vi "纳清pH电极校准.vi"() -> ()   [LabVIEW 2016, in "斯坦道多参数.lvlib"]
uses:
  <vilib>/Utility/miscctls.llb/LVPointTypeDef.ctl
  <vilib>/Analysis/NI_AALBase.lvlib
panel:
  out "滤波设定":sgl
  out "第二点信号值":dbl
  out "第一点信号值":dbl
  out "报警信息":string
  out "通讯状态":string
  out "第二点校准值":dbl
  out "第一点校准值":dbl
  in  "校准停止":bool
  in  "校准启动":bool
  in  "校准模式":u16(ring) items=["两点校准", "单点校准"]
  out "最小值":sgl format="%#.2f"
  out "最大值":sgl format="%#.2f"
  out "波形图表":dbl(graph) caption="历史曲线"
  out "mean":dbl caption="均值" format="%#.2f"
  out "standard deviation":dbl caption="标准差" format="%#.2f"
  out "变异系数":dbl format="%#.6f"
  out "测量值":sgl format="%#.2f"
  out "提示":string
  out "标液2":sgl
  out "标液1":sgl
  out "原始光强数值":sgl caption="信号值" format="%#.6f"
  out "温度":dbl format="%#.2f"
  # "pH电极设定"
  # "℃"
  # "mV"
  # "请选择校准模式:"
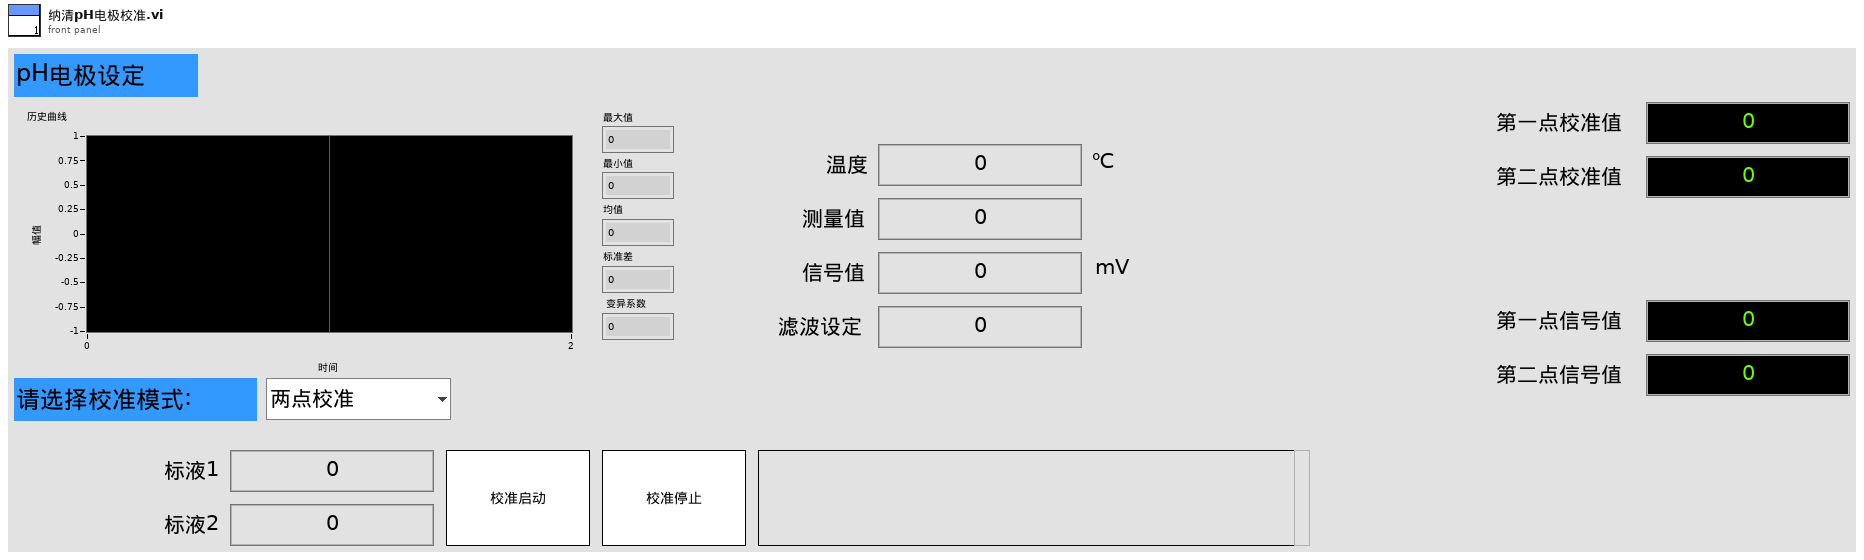
[diagram p1: front panel]
types:
  T1 = enum16{"pH", "DO", "Cond", "Turb", "ORP", "叶绿素a", "藻密度"}
  T2 = typedef "LVPointTypeDef.ctl" = cluster{"Horizontal":i16, "Vertical":i16}
  T3 = cluster{"报警码":u16, "pH数值":sgl, "0X0003_NC":sgl, "温度数据":sgl, "pH原始信号 mv":sgl, "0X0009_NC":string, "产品名称":string, "序列号":string, "硬件版本":string, "软件版本":string, "通讯地址":u16, "波特率":u16, "设备类型":u16, "0X0026_NC":string, "第一点原始数据":sgl, "第一点校准数据":sgl, "第二点原始数据":sgl, "第二点校准数据":sgl, "探头校准命令":u16, "温度校准参数":sgl, "温度校准命令":u16}
  T4 = cluster{"pH":u32, "DO":u32, "Cond":u32, "Turb":u32, "叶绿素a":u32, "藻密度":u32, "ORP":u32, "COD":u32}
  T5 = enum8{"Enabled", "Disabled", "Disabled and Grayed Out"}
  T6 = cluster{"ph":bool, "DO":bool, "Cond":bool, "Turb":bool, "叶绿素a":bool, "藻密度":bool, "ORP":bool, "COD":bool}
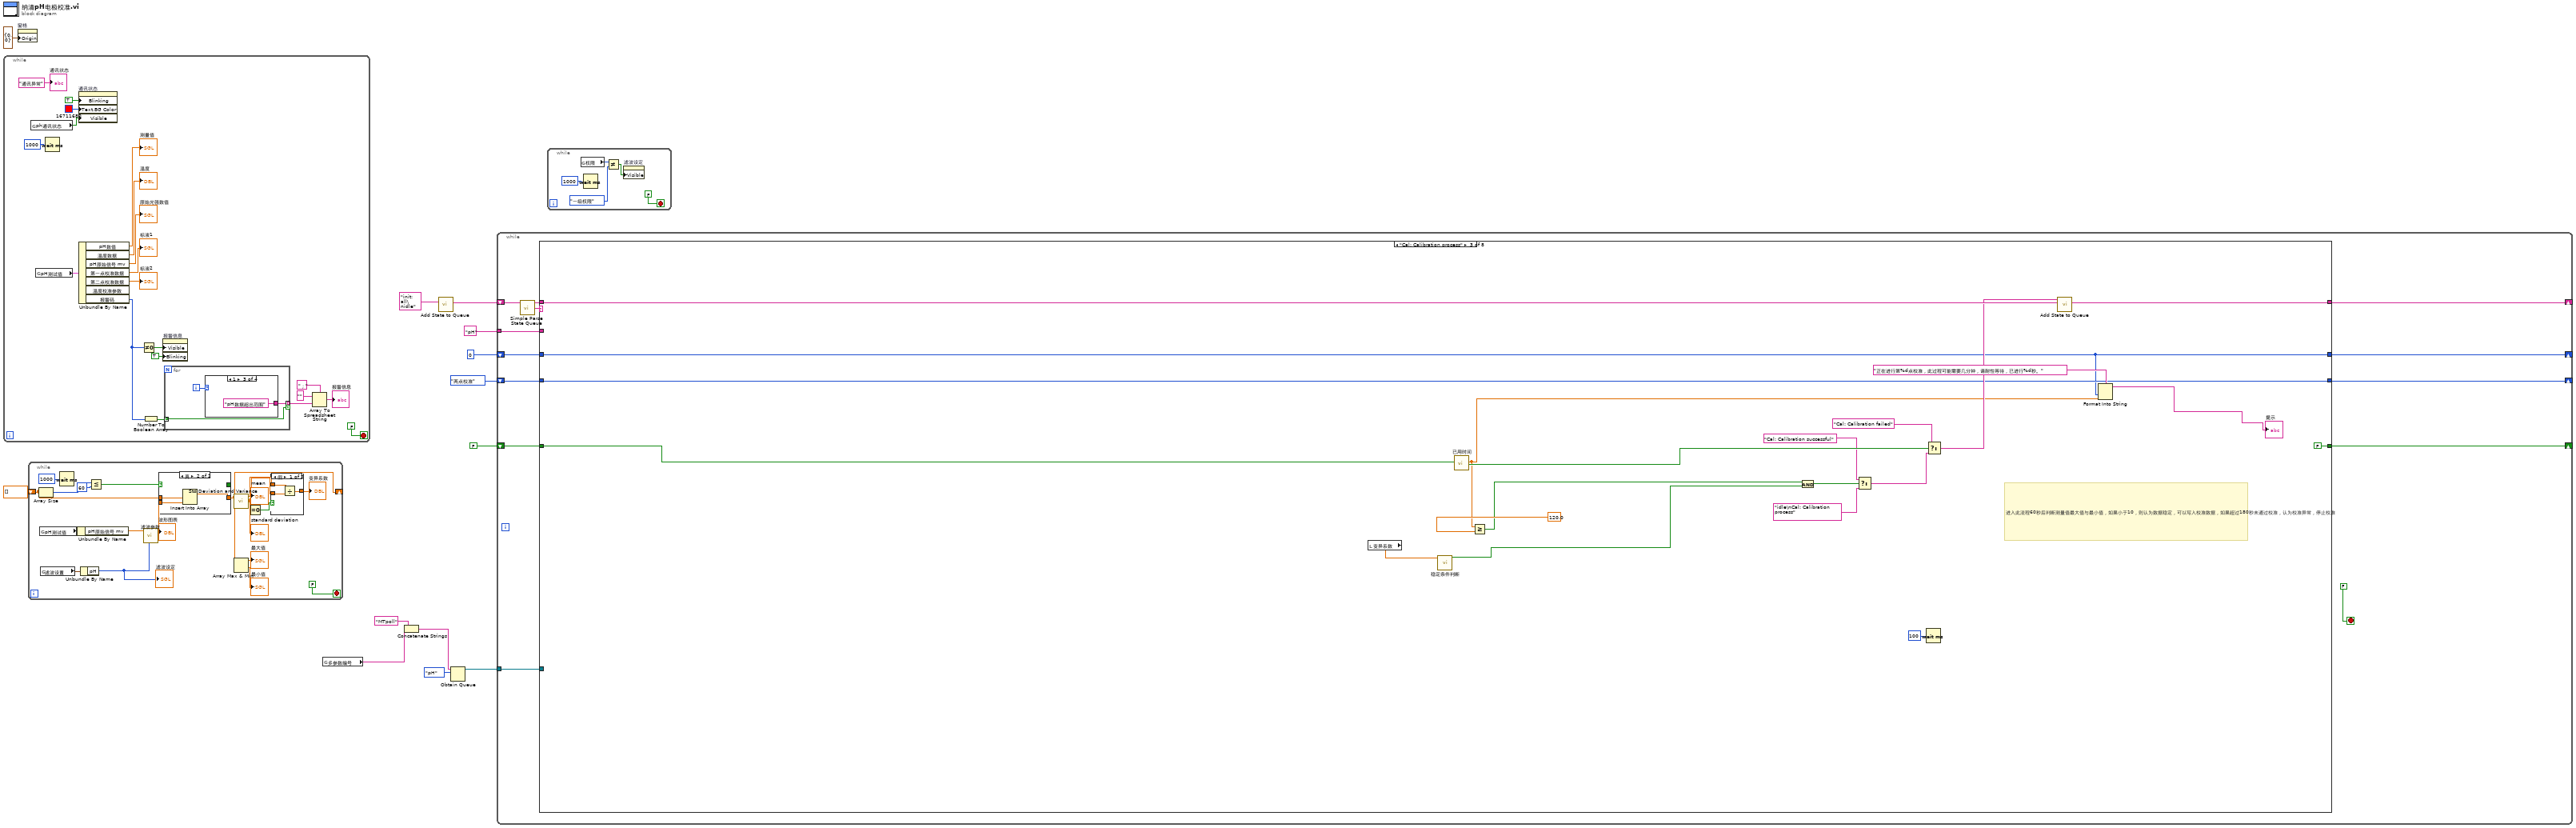
[diagram p0: block diagram]
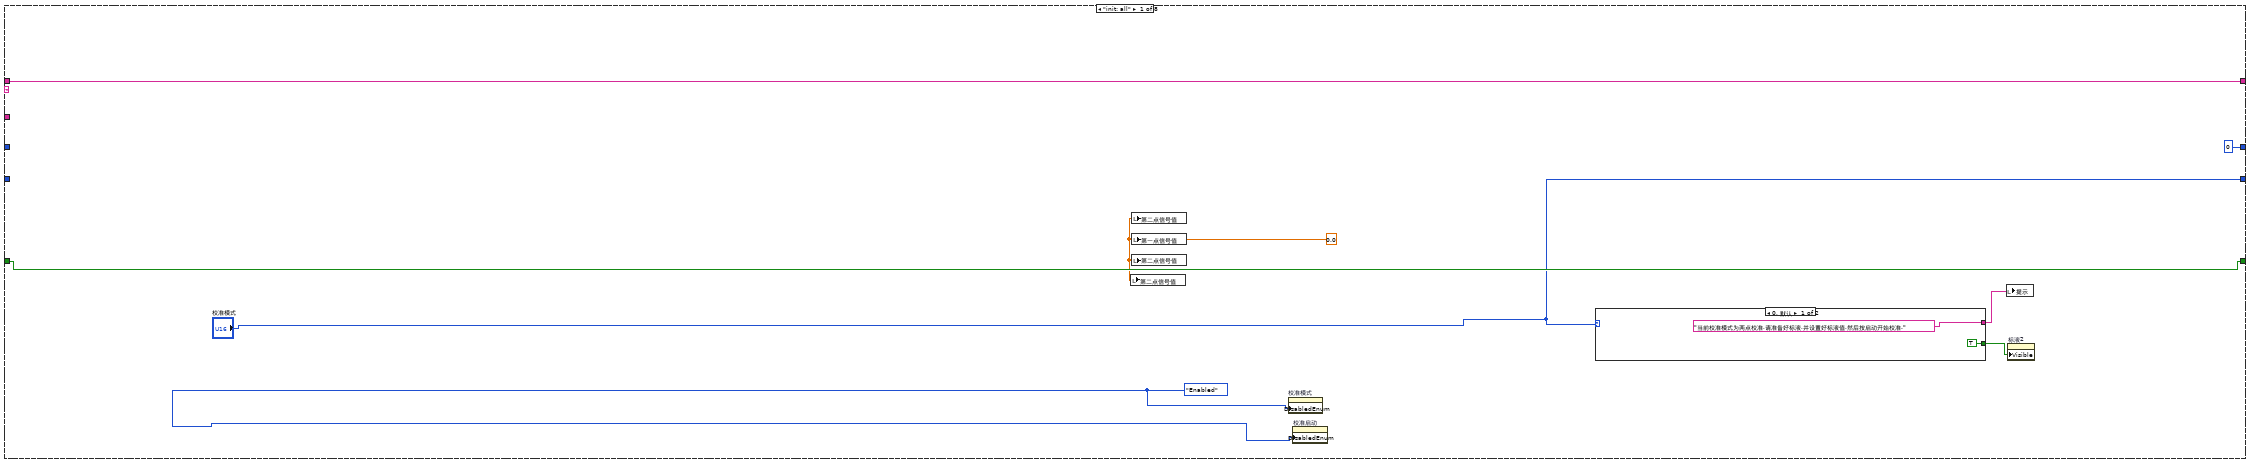
[diagram p2: hidden frame]
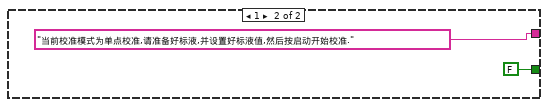
[diagram p3: hidden frame]
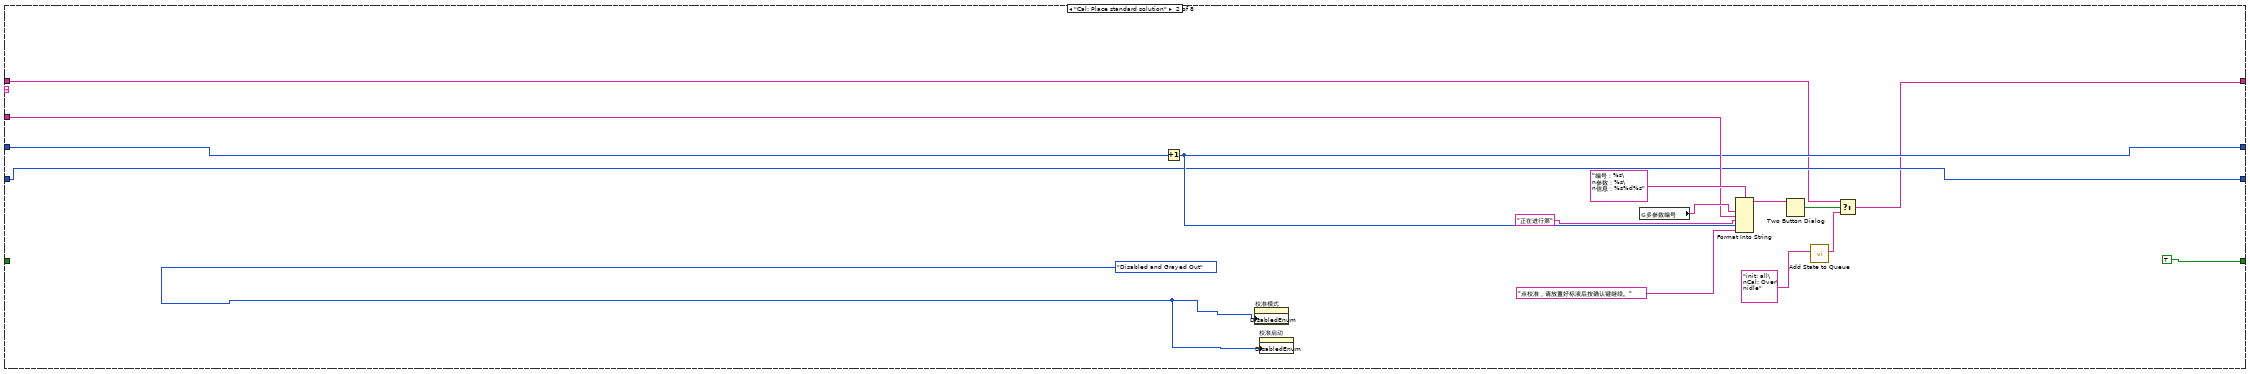
[diagram p4: hidden frame]
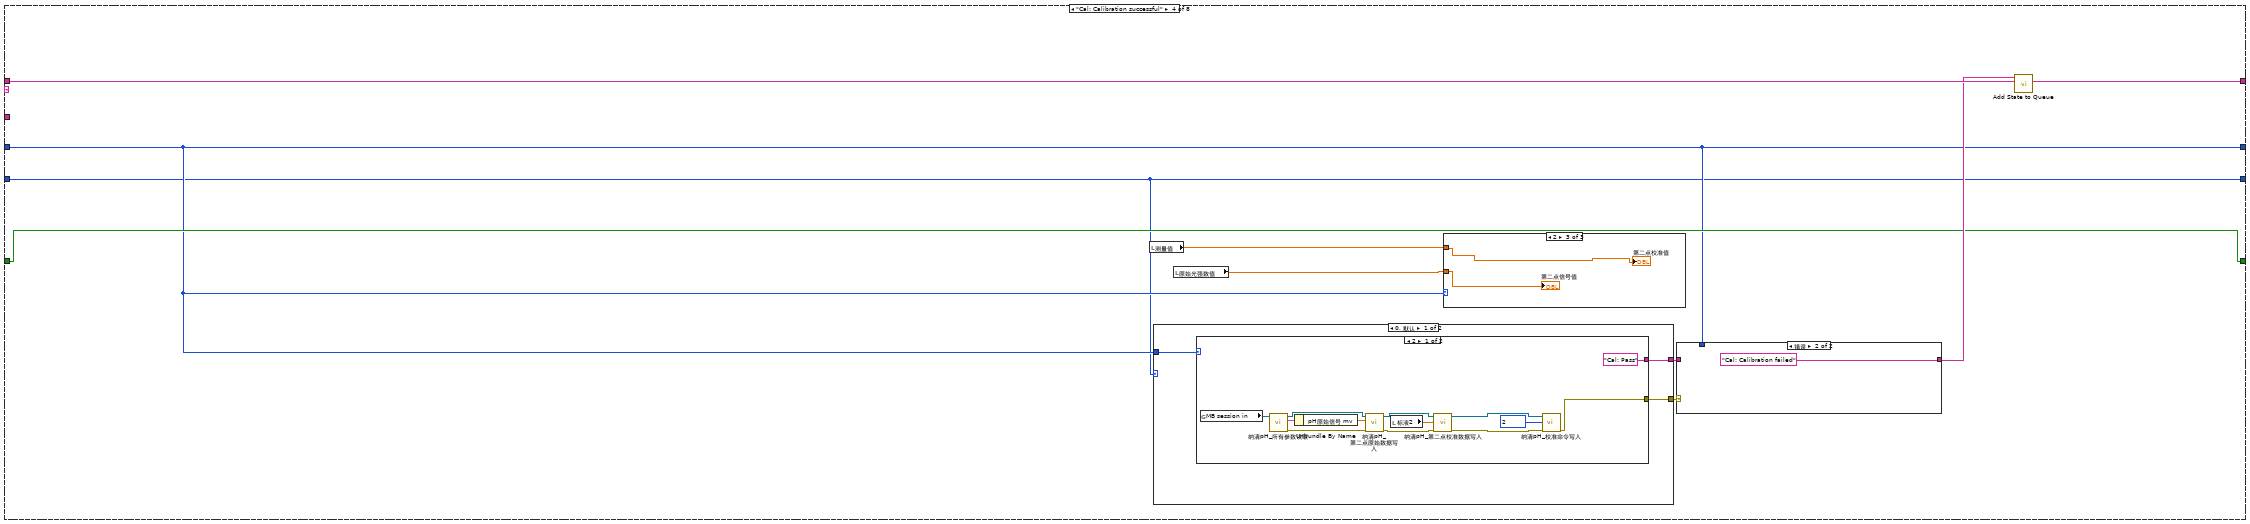
[diagram p5: hidden frame]
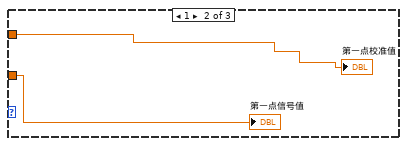
[diagram p7: hidden frame]
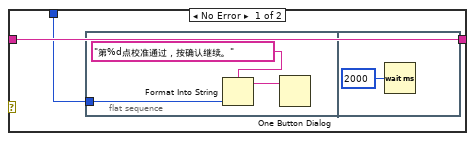
[diagram p8: hidden frame]
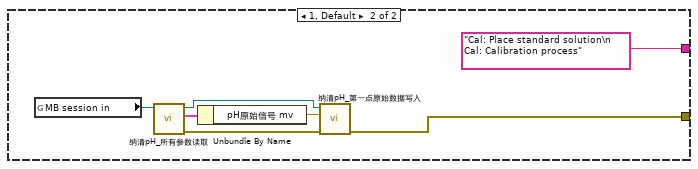
[diagram p9: hidden frame]
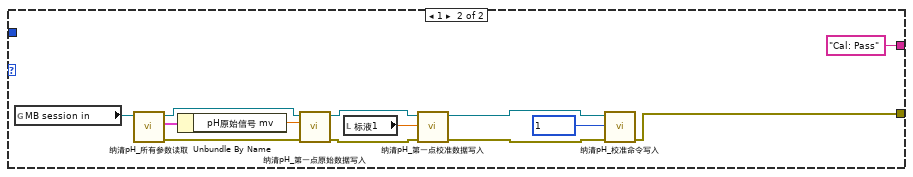
[diagram p10: hidden frame]
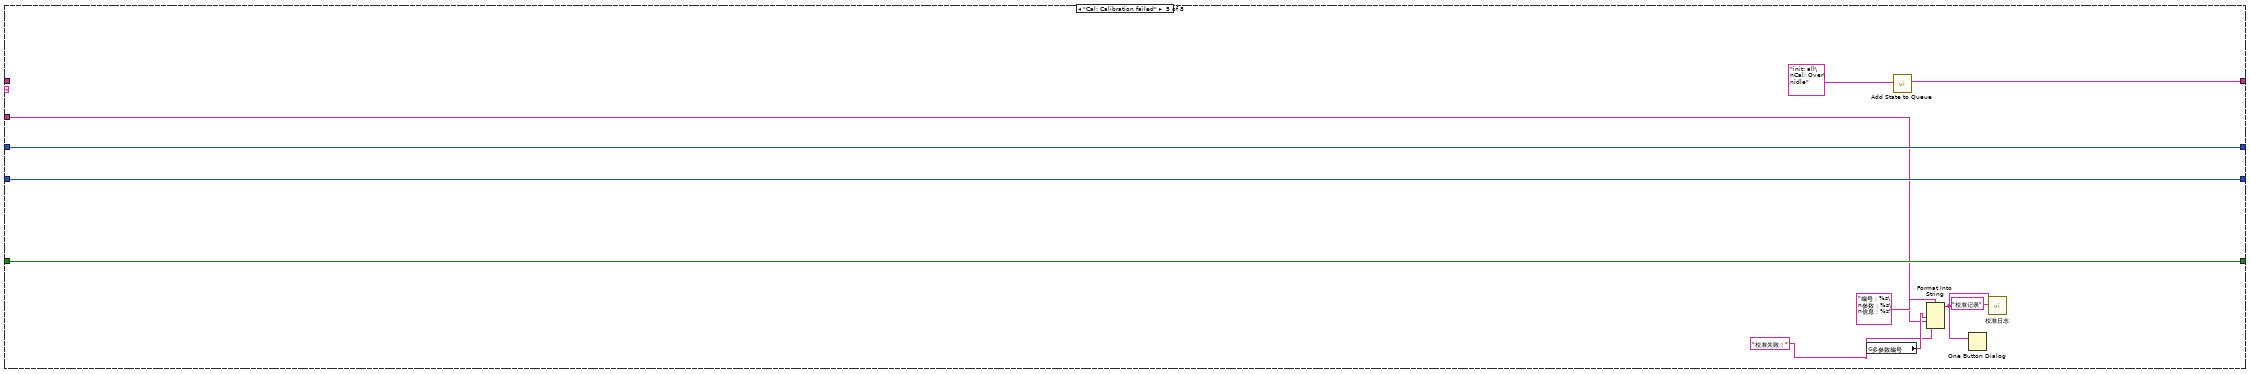
[diagram p11: hidden frame]
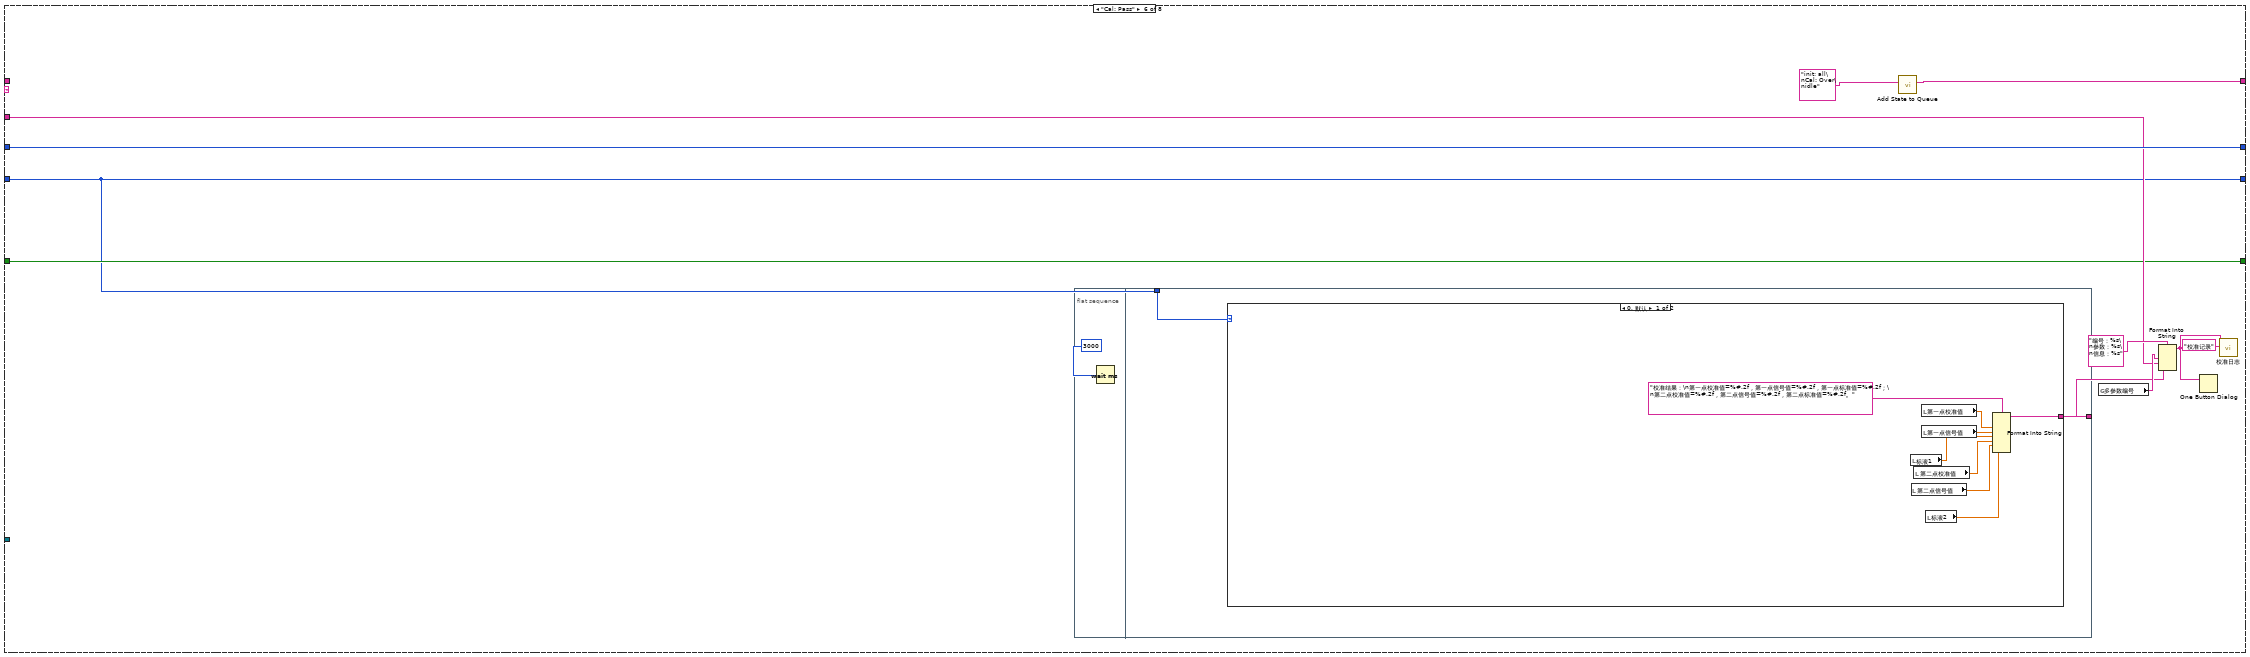
[diagram p12: hidden frame]
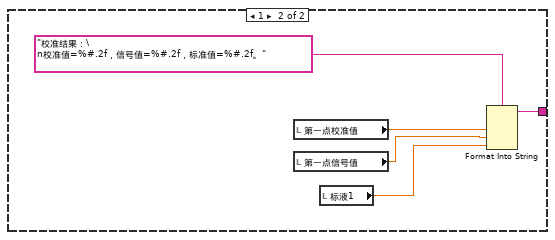
[diagram p13: hidden frame]
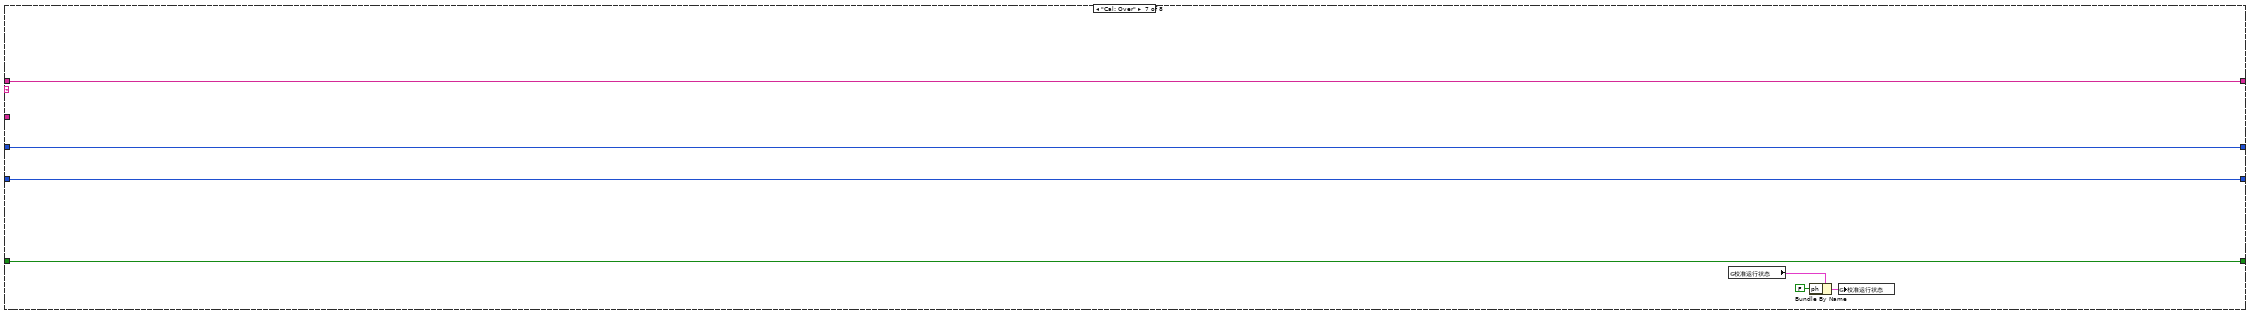
[diagram p14: hidden frame]
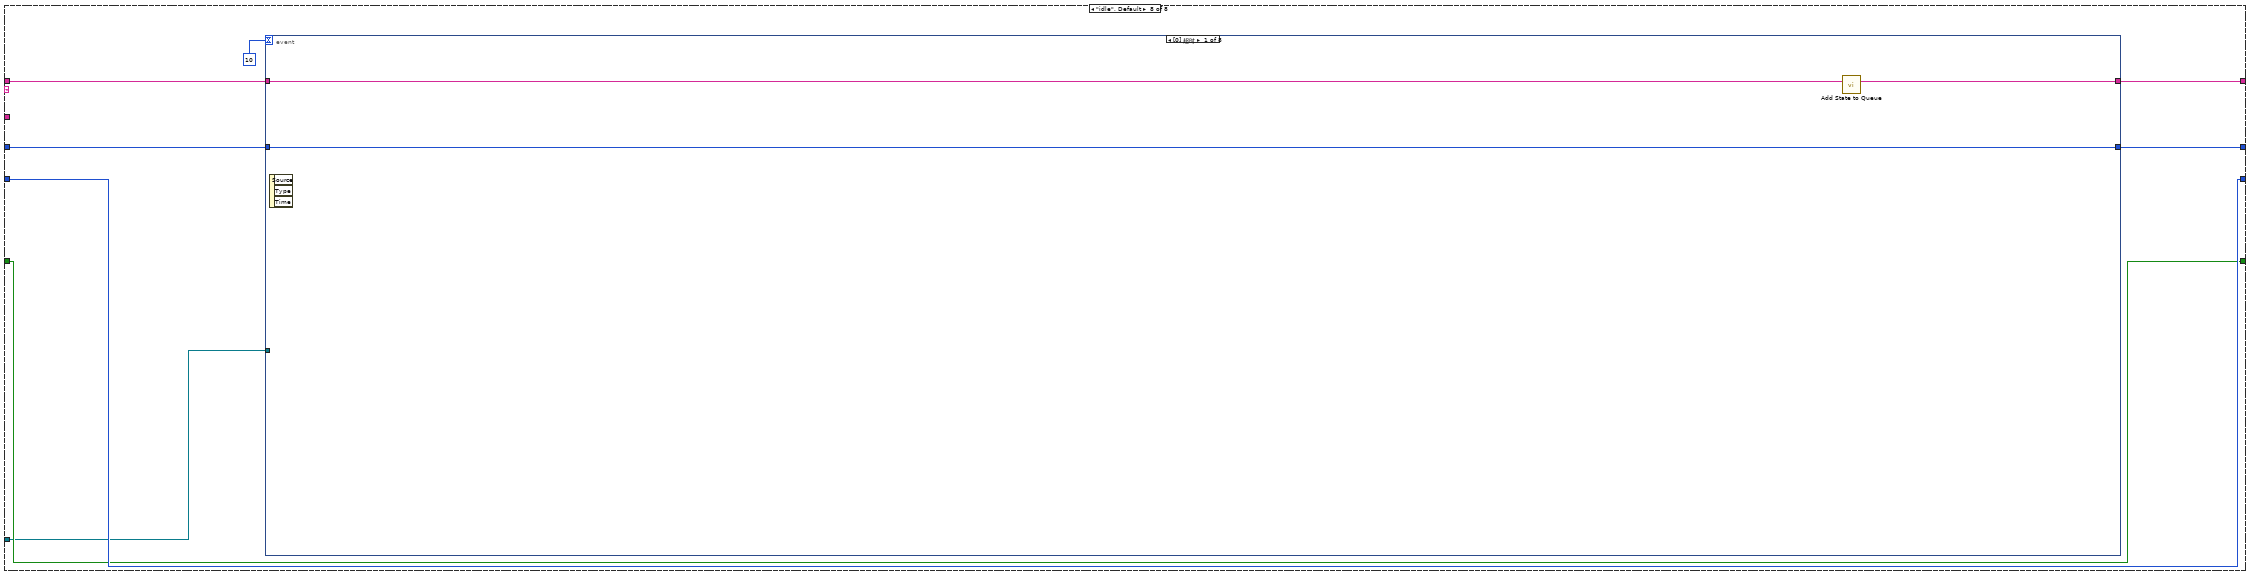
[diagram p15: hidden frame]
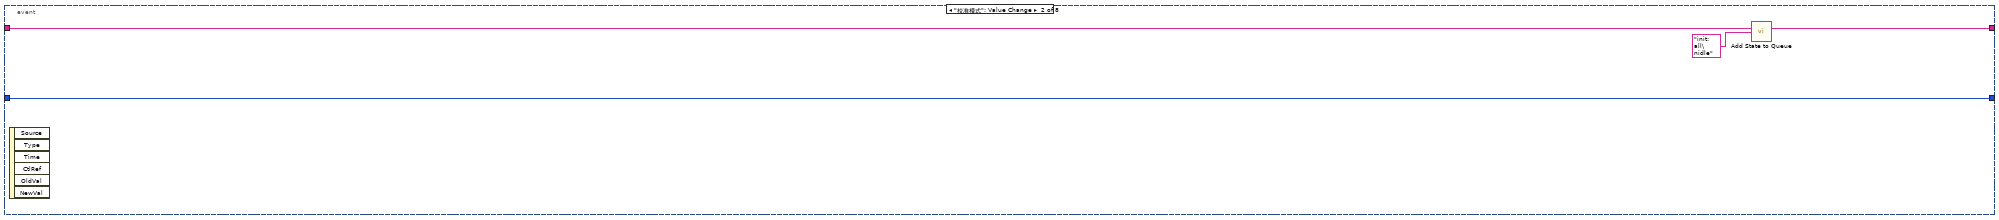
[diagram p16: hidden frame]
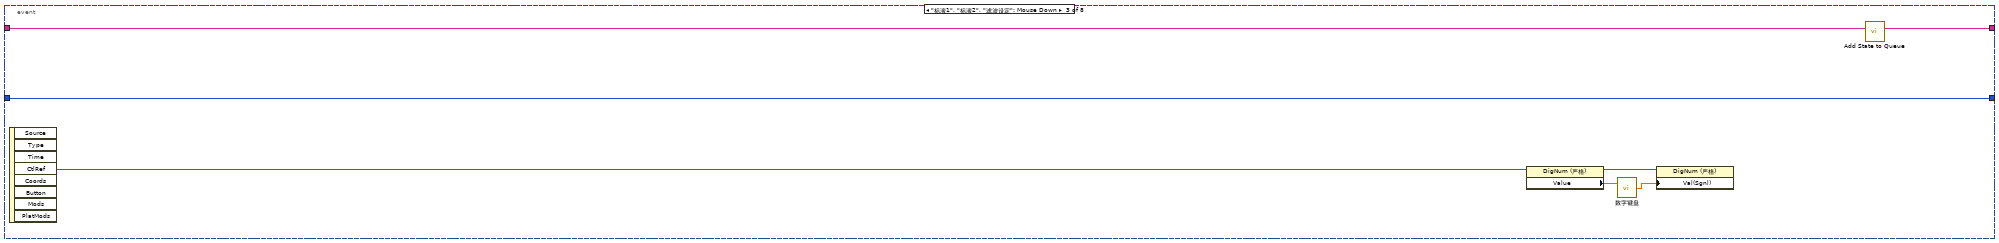
[diagram p17: hidden frame]
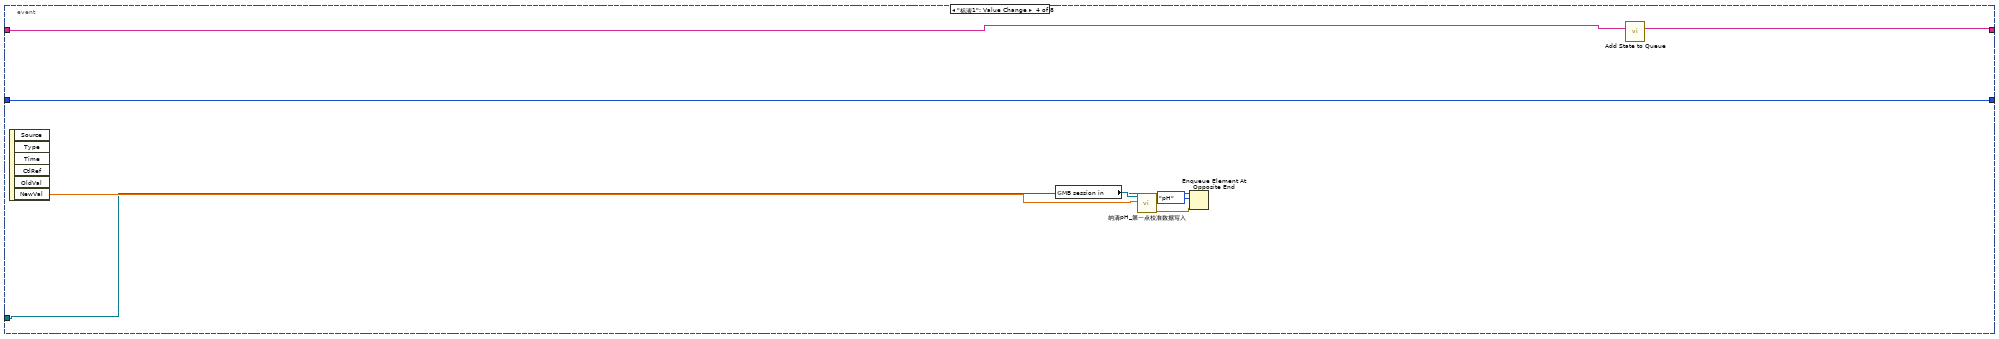
[diagram p18: hidden frame]
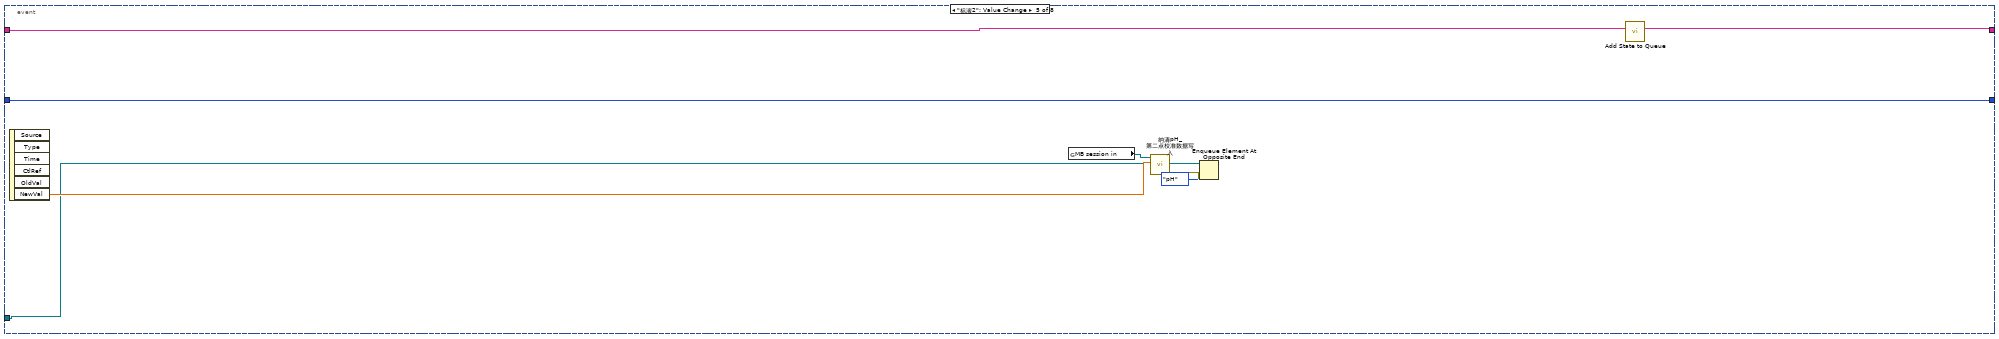
[diagram p19: hidden frame]
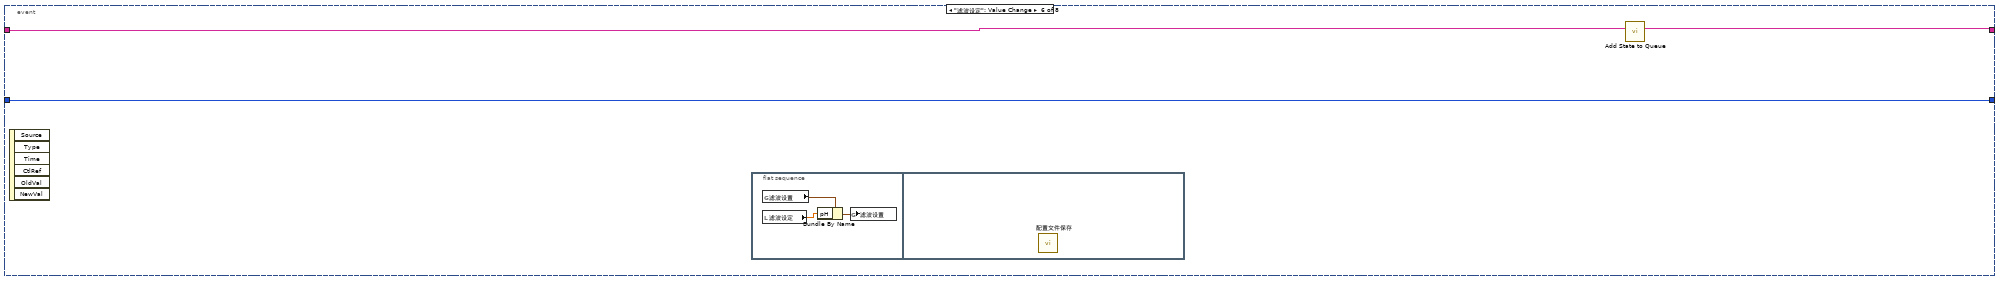
[diagram p20: hidden frame]
diagram:
  n1 = while {
    stop <- FALSE stop-if-true
    n2 = global read "多参数全局变量.vi" "ph通讯状态"() -> (w22:bool)
    n3 = global read "纳清过程全局变量.vi" "pH测试值"() -> (w31:T3)
    n4 = Wait (ms)(milliseconds to wait=u32 1000 ("等待时间（毫秒）")) -> ()  [unwired: 1 out]
    n5 = property on="通讯状态" class="Str"("Blinking"=TRUE ("闪烁"), "Text.BG Color"=u32 16711680, "Visible"=w22) -> ()  [unwired: 2 in, 2 out]
    n6 = Unbundle By Name(w31) -> ("pH数值"=→"测量值":sgl, "温度数据"=→"温度":sgl, "pH原始信号 mv"=→"原始光强数值":sgl, "第一点校准数据"=→"标液1":sgl, "第二点校准数据"=→"标液2":sgl, "报警码"=w16:u16)  [unwired: 1 out]
    n7 = Not Equal To 0?(x=w16) -> (x != 0?=w15:bool)
    n8 = Number To Boolean Array(number=w16) -> (Boolean array=w21:bool[])
    n9 = property on="报警信息" class="Str"("Visible"=w15, "Blinking"=TRUE ("闪烁")) -> ()  [unwired: 2 in, 2 out]
    n10 = for {
      tunnel: w21 -> [w34] mode=indexing
      tunnel: [w35] -> w20 mode=indexing if=w34
      i -> [w36]
      n11 = case shown="1" w36 {
        tunnel: [_ "温度超出范围" "pH数据超出范围" "温度传感器故障"] -> w35
        frame Default {
        }
        frame 0 {
        }
        frame 1 {
        }
        frame 8 {
        }
      }
    }
    n12 = Array To Spreadsheet String(delimiter (Tab)="；" ("分隔符(Tab)"), array=w20, 3:"" ("格式字符串")) -> (spreadsheet string=→"报警信息":string)
    "通讯状态" <- "通讯异常" ("当前串口")
  }
  n13 = property on="窗格" class="Pane"("Origin"=T2 {"Horizontal"=0, "Vertical"=0} ("原点")) -> ()  [unwired: 2 in, 2 out]
  n14 = while {
    shift-right: [w47] -> _
    shift-left: sgl[] [] -> [w53]
    stop <- FALSE stop-if-true
    n15 = Array Size(array=w53) -> (size(s)=w55:i32)
    n16 = global read "纳清过程全局变量.vi" "pH测试值"() -> (w44:T3)
    n17 = global read "断电保存变量.vi" "滤波设置"() -> (w41:T4)
    n18 = Wait (ms)(milliseconds to wait=u32 1000 ("等待时间（毫秒）")) -> ()  [unwired: 1 out]
    n19 = Unbundle By Name(w44) -> ("pH原始信号 mv"=w43:sgl)
    n20 = Unbundle By Name(w41) -> ("pH"=w40:u32)
    "滤波设定" <- w40
    n21 = Less Or Equal?(x=w55, y=60) -> (x <= y?=w54:bool)
    n22 = call "滤波参数.vi"("滤波次数"=w40, "x"=w43) -> ("mode"=w42:dbl)  [unwired: 9 in]
    "波形图表" <- w42
    n23 = case shown="真" w54 {
      tunnel: w53 -> [w66 w69]
      tunnel: w42 -> [w64 w68]
      tunnel: [w62 w67] -> w47
      tunnel: [TRUE _] -> _
      frame False {
        n24 = Replace Array Subset(array=w66, new element=w64) -> (w65:sgl[])  [unwired: 1 in]
        n25 = Rotate 1D Array(1:w65, 2:-1 ("n")) -> (0:w62:sgl[])
      }
      frame True {
        n26 = Insert Into Array(array=w69, new element=w68) -> (w67:sgl[])  [unwired: 1 in]
      }
    }
    n27 = call <vilib>:"Std Deviation and Variance.vi"("X"=w47) -> ("mean"=w51:dbl, "standard deviation"=w50:dbl)  [unwired: 1 in, 1 out]
    "mean" <- w51
    "standard deviation" <- w50
    n28 = Array Max & Min(array=w47) -> (max value=→"最大值":sgl, min value=→"最小值":sgl)  [unwired: 2 out]
    n29 = Equal To 0?(x=w51) -> (x = 0?=w52:bool)
    n30 = case shown="假" w52 {
      tunnel: w50 -> [w60 _]
      tunnel: [w59 _] -> w49
      tunnel: w51 -> [w58 _]
      frame False {
        n31 = Divide(x=w60, y=w58) -> (x/y=w59:dbl)
      }
      frame True {
      }
    }
    "变异系数" <- w49
  }
  n32 = global read "多参数全局变量.vi" "多参数编号"() -> (w2:string)
  n33 = Concatenate Strings("MTpoll" ("名称（未命名）"), w2) -> (w4:string)
  n34 = call "Add State to Queue.vi"("State(s) In (\"\")"="init: all\nidle" ("State(s) In (\"\")")) -> ("States Out"=w10:string)  [unwired: 14 in]
  n35 = Obtain Queue(name (unnamed)=w4, element data type=T1."pH" ("枚举")) -> (queue out=w1:refnum<queue>)  [unwired: 3 in, 2 out]
  n36 = while {
    shift-right: [w78] -> _
    shift-left: w10 -> [w82]
    shift-right: [w75] -> _
    shift-left: 0 -> [w77]
    tunnel: "pH" ("State(s) In (\"\")") -> [w76]
    shift-right: [w73] -> _
    shift-left: enum16{"两点校准", "单点校准"}."两点校准" ("校准模式") -> [w74]
    shift-right: [w71] -> _
    shift-left: FALSE -> [w72]
    tunnel: w1 -> [w70]
    stop <- FALSE stop-if-true
    n37 = call "Simple Parse State Queue.vi"("State Queue"=w82) -> ("Remain States"=w79:string, "Next State"=w80:string)  [unwired: 13 in]
    n38 = case shown="\"Cal: Calibration process\"" w80 {
      tunnel: w79 -> [w90 w98 w130 w139 _ _ w233 w241]
      tunnel: [w90 w97 w129 w138 w196 w201 w233 w240] -> w78
      tunnel: w77 -> [_ w106 w115 w133 w199 w210 w232 w238]
      tunnel: w76 -> [_ w107 _ _ w190 w206 _ _]
      tunnel: [0 w104 w115 w133 w199 w210 w232 w239] -> w75
      tunnel: w74 -> [_ w103 w116 w132 w198 w202 w231 w237]
      tunnel: ["校准模式" w103 w116 w132 w198 w202 w231 w237] -> w73
      tunnel: w72 -> [w87 _ w118 w134 w197 w205 w230 w235]
      tunnel: [w87 TRUE FALSE w134 w197 w205 w230 w235] -> w71
      tunnel: w70 -> [_ _ _ _ _ _ _ w234]
      frame "init: all" {
        w85 = T5."Enabled" ("禁用")
        w86 = 0.0 ("第一点校准值")
        n39 = local write "第二点信号值"(w86) -> ()
        n40 = local write "第二点信号值"(w86) -> ()
        n41 = local write "第一点信号值"(w86) -> ()
        n42 = local write "第二点信号值"(w86) -> ()
        n43 = property on="校准模式" class="Ring (严格)"("DisabledEnum"=w85) -> ()  [unwired: 2 in, 2 out]
        n44 = property on="校准启动" class="Bool"("DisabledEnum"=w85) -> ()  [unwired: 2 in, 2 out]
        n45 = case shown="0, 默认" "校准模式" {
          tunnel: ["当前校准模式为两点校准,请准备好标液,并设置好标液值,然后按启动开始校准." ("提示") "当前校准模式为单点校准,请准备好标液,并设置好标液值,然后按启动开始校准." ("提示")] -> w89
          tunnel: [TRUE ("可见") FALSE ("可见")] -> w83
          frame 0, Default {
          }
          frame 1 {
          }
        }
        n46 = local write "提示"(w89) -> ()
        n47 = property on="标液2" class="DigNum (严格)"("Visible"=w83) -> ()  [unwired: 2 in, 2 out]
      }
      frame "Cal: Place standard solution" {
        w96 = T5."Disabled and Grayed Out" ("禁用")
        n48 = Increment(x=w106) -> (x+1=w104:i32)
        n49 = property on="校准模式" class="Ring (严格)"("DisabledEnum"=w96) -> ()  [unwired: 2 in, 2 out]
        n50 = property on="校准启动" class="Bool"("DisabledEnum"=w96) -> ()  [unwired: 2 in, 2 out]
        n51 = global read "多参数全局变量.vi" "多参数编号"() -> (w109:string)
        n52 = Format Into String(format string="编号：%s\n参数：%s\n信息：%s%d%s" ("格式字符串"), w109, w107, "正在进行第" ("消息"), w104, "点校准，请放置好标液后按确认键继续。" ("消息")) -> (resulting string=w101:string)  [unwired: 2 in, 1 out]
        n53 = Two Button Dialog(message=w101) -> (T button?=w100:bool)  [unwired: 2 in]
        n54 = call "Add State to Queue.vi"("State(s) In (\"\")"="init: all\nCal: Over\nidle" ("State(s) In (\"\")")) -> ("States Out"=w99:string)  [unwired: 14 in]
        n55 = Select(t=w98, s=w100, f=w99) -> (s? t:f=w97:string)
      }
      frame "Cal: Calibration process" {
        # "进入此流程60秒后判断测量值最大值与最小值，如果小于10，则认为数据稳定，可以写入校准数据，如果超过180秒未通过校准，认为校准异常，停止校准"
        n56 = local read "变异系数"() -> (w112:dbl)
        n57 = call "稳定条件判断.vi"("变异系数"=w112) -> ("布尔"=w111:bool)  [unwired: 10 in]
        n58 = call "已用时间"("Reset"=w118) -> ("Elapsed Time (s)"=w114:dbl, "Time has Elapsed"=w131:bool)  [unwired: 11 in, 6 out]
        n59 = Greater Or Equal?(x=w114, y=120.0) -> (x >= y?=w126:bool)
        n60 = And(x=w126, y=w111) -> (x .and. y?=w123:bool)
        n61 = Select(t="Cal: Calibration successful" ("State(s) In (\"\")"), s=w123, f="idle\nCal: Calibration process" ("State(s) In (\"\")")) -> (s? t:f=w122:string)
        n62 = Wait (ms)(milliseconds to wait=u32 100 ("等待时间（毫秒）")) -> ()  [unwired: 1 out]
        n63 = Select(t="Cal: Calibration failed" ("State(s) In (\"\")"), s=w131, f=w122) -> (s? t:f=w121:string)
        n64 = call "Add State to Queue.vi"("State(s) In Front (\"\")"=w121, "State(s) In (\"\")"=w130) -> ("States Out"=w129:string)  [unwired: 13 in]
        n65 = Format Into String(format string="正在进行第%d点校准，此过程可能需要几分钟，请耐性等待，已进行%d秒。" ("格式字符串"), w115, w114) -> (resulting string=→"提示":string)  [unwired: 2 in, 1 out]
      }
      frame "Cal: Calibration successful" {
        n66 = local read "测量值"() -> (w135:sgl)
        n67 = case shown="0, 默认" w132 {
          tunnel: [w155 w176] -> w141
          tunnel: [w154 "Cal: Pass" ("State(s) In (\"\")")] -> w140
          tunnel: w133 -> [w153 _]
          frame 0, Default {
            n68 = case shown="2" w153 {
              tunnel: [w156 w169] -> w155
              tunnel: ["Cal: Pass" ("State(s) In (\"\")") "Cal: Place standard solution\n Cal: Calibration process" ("State(s) In (\"\")")] -> w154
              frame 2 {
                n69 = global read "多参数全局变量.vi" "MB session in"() -> (w164:refnum<class "MB_Master.lvclass">)
                n70 = call "纳清pH_所有参数读取.vi"("MB session in"=w164) -> ("error out"=w166:errorcluster, "输出值"=w163:T3, "MB session out"=w165:refnum<class "MB_Master.lvclass">)  [unwired: 8 in]
                n71 = Unbundle By Name(w163) -> ("pH原始信号 mv"=w162:sgl)
                n72 = call "纳清pH_第二点原始数据写入.vi"("error in (no error)"=w166, "数值"=w162, "MB session in"=w165) -> ("error out"=w161:errorcluster, "MB session out"=w160:refnum<class "MB_Master.lvclass">)  [unwired: 7 in]
                n73 = local read "标液2"() -> (w157:sgl)
                n74 = call "纳清pH_第二点校准数据写入.vi"("error in (no error)"=w161, "数值"=w157, "MB session in"=w160) -> ("error out"=w159:errorcluster, "MB session out"=w158:refnum<class "MB_Master.lvclass">)  [unwired: 7 in]
                n75 = call "纳清pH_校准命令写入.vi"("error in (no error)"=w159, "数值"=u16 2 ("starting address"), "MB session in"=w158) -> ("error out"=w156:errorcluster)  [unwired: 7 in, 1 out]
              }
              frame 1, Default {
                n76 = global read "多参数全局变量.vi" "MB session in"() -> (w172:refnum<class "MB_Master.lvclass">)
                n77 = call "纳清pH_所有参数读取.vi"("MB session in"=w172) -> ("error out"=w174:errorcluster, "输出值"=w171:T3, "MB session out"=w173:refnum<class "MB_Master.lvclass">)  [unwired: 8 in]
                n78 = Unbundle By Name(w171) -> ("pH原始信号 mv"=w170:sgl)
                n79 = call "纳清pH_第一点原始数据写入.vi"("error in (no error)"=w174, "数值"=w170, "MB session in"=w173) -> ("error out"=w169:errorcluster)  [unwired: 7 in, 1 out]
              }
            }
          }
          frame 1 {
            n80 = global read "多参数全局变量.vi" "MB session in"() -> (w184:refnum<class "MB_Master.lvclass">)
            n81 = call "纳清pH_所有参数读取.vi"("MB session in"=w184) -> ("error out"=w186:errorcluster, "输出值"=w183:T3, "MB session out"=w185:refnum<class "MB_Master.lvclass">)  [unwired: 8 in]
            n82 = Unbundle By Name(w183) -> ("pH原始信号 mv"=w182:sgl)
            n83 = call "纳清pH_第一点原始数据写入.vi"("error in (no error)"=w186, "数值"=w182, "MB session in"=w185) -> ("error out"=w181:errorcluster, "MB session out"=w180:refnum<class "MB_Master.lvclass">)  [unwired: 7 in]
            n84 = local read "标液1"() -> (w177:sgl)
            n85 = call "纳清pH_第一点校准数据写入.vi"("error in (no error)"=w181, "数值"=w177, "MB session in"=w180) -> ("error out"=w179:errorcluster, "MB session out"=w178:refnum<class "MB_Master.lvclass">)  [unwired: 7 in]
            n86 = call "纳清pH_校准命令写入.vi"("error in (no error)"=w179, "数值"=u16 1 ("starting address"), "MB session in"=w178) -> ("error out"=w176:errorcluster)  [unwired: 7 in, 1 out]
          }
        }
        n87 = local read "原始光强数值"() -> (w136:sgl)
        n88 = case shown="2" w133 {
          tunnel: w136 -> [_ w143 w145]
          tunnel: w135 -> [_ w142 w144]
          frame 0, Default {
          }
          frame 1 {
            "第一点信号值" <- w143
            "第一点校准值" <- w142
          }
          frame 2 {
            "第二点信号值" <- w145
            "第二点校准值" <- w144
          }
        }
        n89 = case shown="错误" w141 {
          tunnel: w140 -> [w147 _]
          tunnel: [w147 "Cal: Calibration failed" ("State(s) In (\"\")")] -> w137
          tunnel: w133 -> [w146 _]
          frame No Error {
            n90 = flat-sequence {
              tunnel: w146 -> [w148]
              frame #0 {
                n91 = Format Into String(format string="第%d点校准通过，按确认继续。" ("格式字符串"), w148) -> (resulting string=w150:string)  [unwired: 2 in, 1 out]
                n92 = One Button Dialog(message=w150) -> ()  [unwired: 1 in, 1 out]
              }
              frame #1 {
                n93 = Wait (ms)(milliseconds to wait=u32 2000 ("等待时间（毫秒）")) -> ()  [unwired: 1 out]
              }
            }
          }
          frame Error {
          }
        }
        n94 = call "Add State to Queue.vi"("State(s) In Front (\"\")"=w137, "State(s) In (\"\")"=w139) -> ("States Out"=w138:string)  [unwired: 13 in]
      }
      frame "Cal: Calibration failed" {
        n95 = global read "多参数全局变量.vi" "多参数编号"() -> (w193:string)
        n96 = call "Add State to Queue.vi"("State(s) In (\"\")"="init: all\nCal: Over\nidle" ("State(s) In (\"\")")) -> ("States Out"=w196:string)  [unwired: 14 in]
        n97 = Format Into String(format string="编号：%s\n参数：%s\n信息：%s" ("格式字符串"), w193, w190, "校准失败！" ("消息")) -> (resulting string=w192:string)  [unwired: 2 in, 1 out]
        n98 = One Button Dialog(message=w192) -> ()  [unwired: 1 in, 1 out]
        n99 = call "校准日志.vi"("table"="校准记录", "日志信息"=w192) -> ()  [unwired: 9 in, 1 out]
      }
      frame "Cal: Pass" {
        n100 = flat-sequence {
          tunnel: [w213] -> w203
          tunnel: w202 -> [w212]
          frame #0 {
            n101 = Wait (ms)(milliseconds to wait=u32 3000 ("等待时间（毫秒）")) -> ()  [unwired: 1 out]
          }
          frame #1 {
            n102 = case shown="0, 默认" w212 {
              tunnel: [w221 w226] -> w213
              frame 0, Default {
                n103 = local read "标液1"() -> (w217:sgl)
                n104 = local read "第二点信号值"() -> (w215:dbl)
                n105 = local read "第二点校准值"() -> (w216:dbl)
                n106 = local read "第一点校准值"() -> (w219:dbl)
                n107 = local read "第一点信号值"() -> (w220:dbl)
                n108 = local read "标液2"() -> (w214:sgl)
                n109 = Format Into String(format string="校准结果：\n第一点校准值=%#.2f，第一点信号值=%#.2f，第一点标准值=%#.2f；\n第二点校准值=%#.2f，第二点信号值=%#.2f，第二点标准值=%#.2f。" ("提示"), w219, w220, w217, w216, w215, w214) -> (resulting string=w221:string)  [unwired: 2 in, 1 out]
              }
              frame 1 {
                n110 = local read "第一点校准值"() -> (w225:dbl)
                n111 = local read "第一点信号值"() -> (w223:dbl)
                n112 = local read "标液1"() -> (w222:sgl)
                n113 = Format Into String(format string="校准结果：\n校准值=%#.2f，信号值=%#.2f，标准值=%#.2f。" ("提示"), w225, w223, w222) -> (resulting string=w226:string)  [unwired: 2 in, 1 out]
              }
            }
          }
        }
        n114 = call "Add State to Queue.vi"("State(s) In (\"\")"="init: all\nCal: Over\nidle" ("State(s) In (\"\")")) -> ("States Out"=w201:string)  [unwired: 14 in]
        n115 = global read "多参数全局变量.vi" "多参数编号"() -> (w207:string)
        n116 = Format Into String(format string="编号：%s\n参数：%s\n信息：%s" ("格式字符串"), w207, w206, w203) -> (resulting string=w204:string)  [unwired: 2 in, 1 out]
        n117 = One Button Dialog(message=w204) -> ()  [unwired: 1 in, 1 out]
        n118 = call "校准日志.vi"("table"="校准记录", "日志信息"=w204) -> ()  [unwired: 9 in, 1 out]
      }
      frame "Cal: Over" {
        n119 = global read "多参数全局变量.vi" "校准运行状态"() -> (w228:T6)
        n120 = Bundle By Name(cluster=w228, "ph"=FALSE) -> (w229:T6)
        n121 = global write "多参数全局变量.vi" "校准运行状态"(w229) -> ()
      }
      frame "idle", Default {
        n122 = event shown="[0] 超时" {
          selector: _ -> [_ _ _ _ _ _ _ _]
          dyn-events: _ -> [_ _ _ _ _ _ _ _]
          timeout: 10 -> [_ _ _ _ _ _ _ _]
          tunnel: w241 -> [w244 w248 w253 w259 w267 w272 w284 _]
          tunnel: [w243 w247 w254 w263 w271 w274 w283 w286] -> w240
          tunnel: [w242 w245 w255 w262 w270 w273 w281 w287] -> w239
          tunnel: w238 -> [w242 w245 w255 w262 w270 w273 w281 w287]
          tunnel: w234 -> [_ _ _ w257 w265 _ _ _]
          event Timeout {
            n123 = event-data() -> ()  [unwired: 1 in, 3 out]
            n124 = call "Add State to Queue.vi"("State(s) In (\"\")"=w244) -> ("States Out"=w243:string)  [unwired: 14 in]
          }
          event "校准模式": Value Change {
            n125 = event-data() -> ()  [unwired: 1 in, 6 out]
            n126 = call "Add State to Queue.vi"("State(s) In (\"\")"=w248, "State(s) At Back (\"\")"="init: all\nidle" ("State(s) In (\"\")")) -> ("States Out"=w247:string)  [unwired: 13 in]
          }
          event "标液1", "标液2", "滤波设定": Mouse Down {
            n127 = event-data() -> ("CtlRef"=w252:refnum<vi>)  [unwired: 1 in, 7 out]
            n128 = property class="DigNum (严格)"(reference=w252) -> (reference out=w249:refnum<vi>, "Value"=w250:sgl)  [unwired: 1 in, 1 out]
            n129 = call "数字键盘.vi"("OldNumber"=w250) -> ("NewNumber"=w251:dbl)  [unwired: 1 in]
            n130 = property class="DigNum (严格)"(reference=w249, "Val(Sgnl)"=w251) -> ()  [unwired: 1 in, 2 out]
            n131 = call "Add State to Queue.vi"("State(s) In (\"\")"=w253) -> ("States Out"=w254:string)  [unwired: 14 in]
          }
          event "标液1": Value Change {
            n132 = event-data() -> ("NewVal"=w260:sgl)  [unwired: 1 in, 5 out]
            n133 = global read "多参数全局变量.vi" "MB session in"() -> (w261:refnum<class "MB_Master.lvclass">)
            n134 = call "纳清pH_第一点校准数据写入.vi"("数值"=w260, "MB session in"=w261) -> ("error out"=w258:errorcluster)  [unwired: 8 in, 1 out]
            n135 = Enqueue Element At Opposite End(queue=w257, element=T1."pH" ("元素"), error in (no error)=w258) -> ()  [unwired: 1 in, 3 out]
            n136 = call "Add State to Queue.vi"("State(s) In (\"\")"=w259) -> ("States Out"=w263:string)  [unwired: 14 in]
          }
          event "标液2": Value Change {
            n137 = event-data() -> ("NewVal"=w268:sgl)  [unwired: 1 in, 5 out]
            n138 = global read "多参数全局变量.vi" "MB session in"() -> (w269:refnum<class "MB_Master.lvclass">)
            n139 = call "纳清pH_第二点校准数据写入.vi"("数值"=w268, "MB session in"=w269) -> ("error out"=w266:errorcluster)  [unwired: 8 in, 1 out]
            n140 = Enqueue Element At Opposite End(queue=w265, element=T1."pH" ("元素"), error in (no error)=w266) -> ()  [unwired: 1 in, 3 out]
            n141 = call "Add State to Queue.vi"("State(s) In (\"\")"=w267) -> ("States Out"=w271:string)  [unwired: 14 in]
          }
          event "滤波设定": Value Change {
            n142 = event-data() -> ()  [unwired: 1 in, 6 out]
            n143 = flat-sequence {
              frame #0 {
                n144 = global read "断电保存变量.vi" "滤波设置"() -> (w277:T4)
                n145 = local read "滤波设定"() -> (w275:sgl)
                n146 = Bundle By Name(cluster=w277, "pH"=w275) -> (w276:T4)
                n147 = global write "断电保存变量.vi" "滤波设置"(w276) -> ()
              }
              frame #1 {
                n148 = call "配置文件保存.vi"() -> ()  [unwired: 12 in]
              }
            }
            n149 = call "Add State to Queue.vi"("State(s) In (\"\")"=w272) -> ("States Out"=w274:string)  [unwired: 14 in]
          }
          event "校准启动": Value Change {
            n150 = event-data() -> ()  [unwired: 1 in, 6 out]
            n151 = global read "多参数全局变量.vi" "校准运行状态"() -> (w279:T6)
            n152 = Bundle By Name(cluster=w279, "ph"=TRUE) -> (w280:T6)
            n153 = global write "多参数全局变量.vi" "校准运行状态"(w280) -> ()
            n154 = call "Add State to Queue.vi"("State(s) In (\"\")"=w284, "State(s) At Back (\"\")"="init: all\nCal: Place standard solution\n Cal: Calibration process\nidle" ("State(s) In (\"\")")) -> ("States Out"=w283:string)  [unwired: 13 in]
          }
          event "校准停止": Value Change {
            n155 = event-data() -> ()  [unwired: 1 in, 6 out]
            n156 = call "Add State to Queue.vi"("State(s) In (\"\")"="init: all\nCal: Over\nidle" ("State(s) In (\"\")")) -> ("States Out"=w286:string)  [unwired: 14 in]
          }
        }
      }
    }
  }
  n157 = while {
    stop <- FALSE stop-if-true
    n158 = global read "多参数全局变量.vi" "权限"() -> (w291:enum16{"一级权限", "二级权限", "三级权限"})
    n159 = Wait (ms)(milliseconds to wait=u32 1000 ("等待时间（毫秒）")) -> ()  [unwired: 1 out]
    n160 = Not Equal?(x=w291, y=enum16{"一级权限", "二级权限", "三级权限"}."一级权限") -> (x != y?=w288:bool)
    n161 = property on="滤波设定" class="DigNum (严格)"("Visible"=w288) -> ()  [unwired: 2 in, 2 out]
  }
